vi "log analysis_gps.vi"() -> ()   [LabVIEW 2018] (continued)
10.7036,22.3000,-0.1718,0.2091,0.0001,-1.383604006,1.084294313,122.725543764,0.4496,0.3001,0.5813,0.1247,0.1017,0.0764,0.1414,0.1471,4.9509,0f000001,0*50e8e3f0\n\t", "DUALANTENNAHEADINGA,USB3,0,49.0,FINESTEERING,2107,282338.100,02000000,d426,15824;SOL_COMPUTED,L1_FLOAT,-1.000000000,82.313255310,23.154996872,0.0,360.000000000,180.000000000,\"631T\",16,5,5,3,04,00,20,01*91a11998\n\t", "DUALANTENNAHEADINGA,USB3,0,50.5,FINESTEERING,2107,282339.100,02008000,d426,15824;INSUFFICIENT_OBS,NONE,0.000000000,0.000000000,0.000000000,0.0,0.000000000,0.000000000,\"\",0,0,0,0,00,00,00,00*9d87d1bd\n\t", "INSPVAXA,USB3,0,52.0,FINESTEERING,2107,282339.650,02008000,471d,15824;INS_ALIGNMENT_COMPLETE,INS_RTKFIXED,37.37060410309,126.72431070985,10.7187,22.3000,-0.1560,0.2044,-0.0028,-0.834208822,1.087221031,121.798208463,0.4988,0.3371,0.6091,0.1298,0.1043,0.0790,0.1415,0.1476,4.9532,0f000001,0*1343af04\n\t", "DUALANTENNAHEADINGA,USB3,0,50.5,FINESTEERING,2107,282340.100,02008000,d426,15824;INSUFFICIENT_OBS,NONE,0.000000000,0.000000000,0.000000000,0.0,0.000000000,0.000000000,\"\",0,0,0,0,00,00,00,00*7b9cfbae\n\t", "DUALANTENNAHEADINGA,USB3,0,50.5,FINESTEERING,2107,282340.600,02008000,d426,15824;INSUFFICIENT_OBS,NONE,0.000000000,0.000000000,0.000000000,0.0,0.000000000,0.000000000,\"\",0,0,0,0,00,00,00,00*d2d79b9f\n\t", "DUALANTENNAHEADINGA,USB3,0,50.5,FINESTEERING,2107,282341.100,02008000,d426,15824;SOL_COMPUTED,NARROW_FLOAT,-1.000000000,114.279808044,-67.503875732,0.0,360.000000000,180.000000000,\"631T\",19,7,7,5,04,00,20,03*2721f886\n\t", "INSPVAXA,USB3,0,51.0,FINESTEERING,2107,282341.650,02008000,471d,15824;INS_ALIGNMENT_COMPLETE,INS_RTKFIXED,37.37060132873,126.72431550625,10.7234,22.3000,-0.1474,0.2047,-0.0035,-0.652632688,1.321187419,121.044830235,0.4988,0.3371,0.6091,0.1298,0.1043,0.0790,0.1415,0.1476,4.9532,0f000001,0*64211db3\n\t", "DUALANTENNAHEADINGA,USB3,0,51.0,FINESTEERING,2107,282342.100,02008000,d426,15824;INSUFFICIENT_OBS,NONE,0.000000000,0.000000000,0.000000000,0.0,0.000000000,0.000000000,\"\",0,0,0,0,00,00,00,00*1fd29d28\n\t", "DUALANTENNAHEADINGA,USB3,0,53.0,FINESTEERING,2107,282342.600,02008000,d426,15824;INSUFFICIENT_OBS,NONE,0.000000000,0.000000000,0.000000000,0.0,0.000000000,0.000000000,\"\",0,0,0,0,00,00,00,00*2c3b97de\n\t", "INSPVAXA,USB3,0,54.0,FINESTEERING,2107,282344.150,02000000,471d,15824;INS_ALIGNMENT_COMPLETE,INS_RTKFIXED,37.37059762700,126.72432213612,10.7457,22.3000,-0.1412,0.2163,0.0072,-0.887257962,1.775723186,120.744197339,0.5693,0.3802,0.6775,0.1345,0.1064,0.0820,0.1423,0.1482,4.9577,0f000001,0*eda97082\n\t", "INSPVAXA,USB3,0,54.0,FINESTEERING,2107,282344.650,02000000,471d,15824;INS_ALIGNMENT_COMPLETE,INS_RTKFIXED,37.37059696338,126.72432331213,10.7485,22.3000,-0.1428,0.2163,0.0073,-0.851471886,1.782877792,120.701591584,0.5693,0.3802,0.6775,0.1345,0.1064,0.0820,0.1423,0.1482,4.9577,0f000001,0*59042419\n\t", "INSPVAXA,USB3,0,55.5,FINESTEERING,2107,282345.150,02000000,471d,15824;INS_ALIGNMENT_COMPLETE,INS_RTKFIXED,37.37059621025,126.72432460307,10.7527,22.3000,-0.1388,0.2123,-0.0024,-0.823739386,1.527099287,120.736340769,0.5930,0.3895,0.7245,0.1352,0.1094,0.0826,0.1432,0.1486,4.9599,0f000001,0*b8434a6e\n\t", "DUALANTENNAHEADINGA,USB3,0,55.5,FINESTEERING,2107,282345.600,02000000,d426,15824;SOL_COMPUTED,L1_FLOAT,-1.000000000,162.531326294,-26.929321289,0.0,360.000000000,180.000000000,\"631T\",14,5,5,5,04,00,20,03*11a6b9e7\n\t", "INSPVAXA,USB3,0,51.0,FINESTEERING,2107,282346.650,02000000,471d,15824;INS_ALIGNMENT_COMPLETE,INS_RTKFIXED,37.37059354728,126.72432896514,10.7808,22.3000,-0.1593,0.2217,0.0028,-1.002740448,1.844752135,120.714031734,0.5188,0.3373,0.6687,0.1274,0.1044,0.0789,0.1425,0.1477,4.9597,0f000001,0*e05fc804\n\t", "INSPVAXA,USB3,0,53.5,FINESTEERING,2107,282347.150,02000000,471d,15824;INS_ALIGNMENT_COMPLETE,INS_RTKFIXED,37.37059272987,126.72433032061,10.7898,22.3000,-0.1653,0.2242,0.0071,-0.929787730,1.969126330,120.702008757,0.4813,0.3140,0.6303,0.1252,0.1036,0.0771,0.1422,0.1473,4.9596,0f000001,0*9ccf88c1\n\t", "INSPVAXA,USB3,0,53.5,FINESTEERING,2107,282347.650,02000000,471d,15824;INS_ALIGNMENT_COMPLETE,INS_RTKFIXED,37.37059194697,126.72433163028,10.7970,22.3000,-0.1569,0.2242,0.0124,-0.943778320,2.029286352,120.707003262,0.4813,0.3140,0.6303,0.1252,0.1036,0.0771,0.1422,0.1473,4.9596,0f000001,0*cfe1604c\n\t", "INSPVAXA,USB3,0,51.5,FINESTEERING,2107,282348.650,02000000,471d,15824;INS_ALIGNMENT_COMPLETE,INS_RTKFIXED,37.37059036777,126.72433430477,10.8134,22.3000,-0.1636,0.2313,0.0075,-1.033266783,1.805769894,120.739350596,0.4628,0.3038,0.6031,0.1249,0.1034,0.0763,0.1419,0.1472,4.9599,0f000001,0*467420a2\n\t", "INSPVAXA,USB3,0,51.5,FINESTEERING,2107,282349.650,02000000,471d,15824;INS_ALIGNMENT_COMPLETE,INS_RTKFIXED,37.37058879299,126.72433694056,10.8279,22.3000,-0.1661,0.2333,0.0109,-1.186914388,1.463198419,120.784374977,0.4532,0.2999,0.5832,0.1247,0.1026,0.0761,0.1414,0.1469,4.9608,0f000001,0*9616f401\n\t", "INSPVAXA,USB3,0,52.5,FINESTEERING,2107,282350.150,02000000,471d,15824;INS_ALIGNMENT_COMPLETE,INS_RTKFIXED,37.37058797901,126.72433827202,10.8352,22.3000,-0.1763,0.2301,0.0086,-1.055570073,1.334834507,120.760295852,0.4480,0.2986,0.5686,0.1241,0.1011,0.0762,0.1408,0.1465,4.9619,0f000001,0*f726bccb\n\t", "INSPVAXA,USB3,0,52.5,FINESTEERING,2107,282350.650,02000000,471d,15824;INS_ALIGNMENT_COMPLETE,INS_RTKFIXED,37.37058716740,126.72433957539,10.8417,22.3000,-0.1740,0.2264,0.0121,-0.872298800,1.208067122,120.805643727,0.4480,0.2986,0.5686,0.1241,0.1011,0.0762,0.1408,0.1465,4.9619,0f000001,0*1bc0a6ef\n\t", "INSPVAXA,USB3,0,53.5,FINESTEERING,2107,282351.150,02000000,471d,15824;INS_ALIGNMENT_COMPLETE,INS_RTKFIXED,37.37058636021,126.72434089175,10.8474,22.3000,-0.1737,0.2293,0.0134,-0.911883774,0.960654196,120.863326137,0.4480,0.2986,0.5686,0.1241,0.1011,0.0762,0.1408,0.1465,4.9619,0f000001,0*f3ef71b8\n\t", "INSPVAXA,USB3,0,53.5,FINESTEERING,2107,282351.650,02000000,471d,15824;INS_ALIGNMENT_COMPLETE,INS_RTKFIXED,37.37058558937,126.72434215471,10.8538,22.3000,-0.1759,0.2200,0.0154,-0.934777564,1.004148344,120.872982319,0.4480,0.2986,0.5686,0.1241,0.1011,0.0762,0.1408,0.1465,4.9619,0f000001,0*31170c67\n\t", "INSPVAXA,USB3,0,53.0,FINESTEERING,2107,282352.150,02000000,471d,15824;INS_ALIGNMENT_COMPLETE,INS_RTKFIXED,37.37058479579,126.72434342427,10.8616,22.3000,-0.1887,0.2204,0.0143,-0.790488347,0.999839674,120.821997376,0.4480,0.2986,0.5686,0.1241,0.1011,0.0762,0.1408,0.1465,4.9619,0f000001,0*9c9f2292\n\t", "INSPVAXA,USB3,0,53.0,FINESTEERING,2107,282352.650,02000000,471d,15824;INS_ALIGNMENT_COMPLETE,INS_RTKFIXED,37.37058401212,126.72434466825,10.8699,22.3000,-0.1898,0.2115,0.0109,-0.691065939,1.126816556,120.801550290,0.4480,0.2986,0.5686,0.1241,0.1011,0.0762,0.1408,0.1465,4.9619,0f000001,0*dfeeaeca\n\t", "INSPVAXA,USB3,0,54.5,FINESTEERING,2107,282353.150,02000000,471d,15824;INS_ALIGNMENT_COMPLETE,INS_RTKFIXED,37.37058321062,126.72434596398,10.8773,22.3000,-0.1742,0.2198,0.0094,-0.675574846,1.167497971,120.763135201,0.5451,0.3682,0.6457,0.1338,0.1065,0.0809,0.1421,0.1478,4.9659,0f000001,0*3ed9f220\n\t", "INSPVAXA,USB3,0,54.5,FINESTEERING,2107,282353.650,02000000,471d,15824;INS_ALIGNMENT_COMPLETE,INS_RTKFIXED,37.37058240140,126.72434728277,10.8821,22.3000,-0.1762,0.2174,0.0139,-0.658240149,1.464684464,120.605097651,0.5451,0.3682,0.6457,0.1338,0.1065,0.0809,0.1421,0.1478,4.9659,0f000001,0*55075841\n\t", "INSPVAXA,USB3,0,46.0,FINESTEERING,2107,282354.150,02000000,471d,15824;INS_ALIGNMENT_COMPLETE,INS_RTKFIXED,37.37058158517,126.72434860573,10.8883,22.3000,-0.1761,0.2236,0.0096,-0.460607316,1.517794635,120.410253165,0.4992,0.3307,0.6168,0.1257,0.0997,0.0788,0.1413,0.1466,4.9674,0f000001,0*75609bcc\n\t", "INSPVAXA,USB3,0,46.0,FINESTEERING,2107,282354.650,02000000,471d,15824;INS_ALIGNMENT_COMPLETE,INS_RTKFIXED,37.37058081600,126.72434991701,10.8934,22.3000,-0.1786,0.2176,0.0091,-0.549619810,1.573012469,120.242291746,0.4992,0.3307,0.6168,0.1257,0.0997,0.0788,0.1413,0.1466,4.9674,0f000001,0*21503aba\n\t", "INSPVAXA,USB3,0,52.5,FINESTEERING,2107,282355.150,02000000,471d,15824;INS_ALIGNMENT_COMPLETE,INS_RTKFIXED,37.37058003617,126.72435122954,10.8990,22.3000,-0.1704,0.2109,0.0104,-0.583465901,1.528119993,119.981024145,0.4739,0.3119,0.5957,0.1220,0.0977,0.0777,0.1410,0.1462,4.9689,0f000001,0*126057fe\n\t", "INSPVAXA,USB3,0,52.5,FINESTEERING,2107,282355.650,02000000,471d,15824;INS_ALIGNMENT_COMPLETE,INS_RTKFIXED,37.37057924767,126.72435254533,10.9045,22.3000,-0.1778,0.2238,0.0059,-0.556149260,1.423178014,119.692620317,0.4739,0.3119,0.5957,0.1220,0.0977,0.0777,0.1410,0.1462,4.9689,0f000001,0*50fd9e16\n\t", "INSPVAXA,USB3,0,50.5,FINESTEERING,2107,282356.150,02000000,471d,15824;INS_ALIGNMENT_COMPLETE,INS_RTKFIXED,37.37057847739,126.72435384843,10.9119,22.3000,-0.1686,0.2211,0.0250,-0.610838091,1.352028935,119.375016734,0.4594,0.3023,0.5798,0.1203,0.0972,0.0771,0.1409,0.1459,4.9699,0f000001,0*f72577eb\n\t", "INSPVAXA,USB3,0,50.5,FINESTEERING,2107,282356.650,02000000,471d,15824;INS_ALIGNMENT_COMPLETE,INS_RTKFIXED,37.37057772160,126.72435517265,10.9178,22.3000,-0.1723,0.2271,0.0230,-0.636591933,1.172282791,119.120900603,0.4594,0.3023,0.5798,0.1203,0.0972,0.0771,0.1409,0.1459,4.9699,0f000001,0*423d8117\n\t", "INSPVAXA,USB3,0,52.0,FINESTEERING,2107,282357.150,02000000,471d,15824;INS_ALIGNMENT_COMPLETE,INS_RTKFIXED,37.37057699183,126.72435647012,10.9247,22.3000,-0.1655,0.2123,0.0266,-0.635674987,1.199232102,118.840756157,0.4503,0.2976,0.5676,0.1194,0.0970,0.0768,0.1408,0.1458,4.9705,0f000001,0*6596f8d2\n\t", "INSPVAXA,USB3,0,52.0,FINESTEERING,2107,282357.650,02000000,471d,15824;INS_ALIGNMENT_COMPLETE,INS_RTKFIXED,37.37057627543,126.72435778684,10.9314,22.3000,-0.1654,0.2174,0.0126,-0.648643975,1.318562977,118.602215065,0.4503,0.2976,0.5676,0.1194,0.0970,0.0768,0.1408,0.1458,4.9705,0f000001,0*56e0c8f4\n\t", "INSPVAXA,USB3,0,49.0,FINESTEERING,2107,282358.150,02000000,471d,15824;INS_ALIGNMENT_COMPLETE,INS_RTKFIXED,37.37057556621,126.72435909816,10.9380,22.3000,-0.1614,0.2140,0.0160,-0.816236405,1.456902249,118.427735128,0.4453,0.2956,0.5586,0.1188,0.0967,0.0767,0.1406,0.1456,4.9710,0f000001,0*b637b657\n\t", "INSPVAXA,USB3,0,49.0,FINESTEERING,2107,282358.650,02000000,471d,15824;INS_ALIGNMENT_COMPLETE,INS_RTKFIXED,37.37057483953,126.72436042274,10.9431,22.3000,-0.1620,0.2072,0.0216,-0.840006247,1.481756490,118.251827857,0.4453,0.2956,0.5586,0.1188,0.0967,0.0767,0.1406,0.1456,4.9710,0f000001,0*14500fa5\n\t", "INSPVAXA,USB3,0,50.0,FINESTEERING,2107,282359.150,02000000,471d,15824;INS_ALIGNMENT_COMPLETE,INS_RTKFIXED,37.37057411290,126.72436171376,10.9480,22.3000,-0.1710,0.2086,0.0288,-0.732849795,1.756620997,118.132387326,0.4424,0.2949,0.5520,0.1182,0.0959,0.0768,0.1404,0.1455,4.9710,0f000001,0*33ffa9dc\n\t", "INSPVAXA,USB3,0,50.0,FINESTEERING,2107,282359.650,02000000,471d,15824;INS_ALIGNMENT_COMPLETE,INS_RTKFIXED,37.37057338322,126.72436305467,10.9529,22.3000,-0.1728,0.2229,0.0180,-0.801068797,1.536454287,118.115818478,0.4424,0.2949,0.5520,0.1182,0.0959,0.0768,0.1404,0.1455,4.9710,0f000001,0*c3454afa\n\t", "INSPVAXA,USB3,0,48.5,FINESTEERING,2107,282360.150,02000000,471d,15824;INS_ALIGNMENT_COMPLETE,INS_RTKFIXED,37.37057265059,126.72436438219,10.9582,22.3000,-0.1754,0.2257,0.0186,-0.842848206,1.417409471,118.070069819,0.4412,0.2945,0.5472,0.1174,0.0950,0.0769,0.1402,0.1453,4.9710,0f000001,0*6a16ee00\n\t", "INSPVAXA,USB3,0,48.5,FINESTEERING,2107,282360.650,02000000,471d,15824;INS_ALIGNMENT_COMPLETE,INS_RTKFIXED,37.37057191747,126.72436570845,10.9626,22.3000,-0.1784,0.2288,0.0199,-0.831650114,1.387719615,118.066694933,0.4412,0.2945,0.5472,0.1174,0.0950,0.0769,0.1402,0.1453,4.9710,0f000001,0*684747fc\n\t", "INSPVAXA,USB3,0,48.0,FINESTEERING,2107,282361.650,02000000,471d,15824;INS_ALIGNMENT_COMPLETE,INS_RTKFIXED,37.37057042530,126.72436839921,10.9712,22.3000,-0.1758,0.2244,0.0130,-0.782174586,1.064389692,118.205019127,0.4403,0.2942,0.5440,0.1166,0.0940,0.0770,0.1401,0.1452,4.9712,0f000001,0*a289776d\n\t", "INSPVAXA,USB3,0,52.0,FINESTEERING,2107,282362.150,02000000,471d,15824;INS_ALIGNMENT_COMPLETE,INS_RTKFIXED,37.37056968661,126.72436971158,10.9754,22.3000,-0.1789,0.2227,0.0149,-0.712007512,1.145542222,118.217293959,0.4394,0.2937,0.5418,0.1158,0.0932,0.0771,0.1400,0.1450,4.9721,0f000001,0*3affd318\n\t", "INSPVAXA,USB3,0,52.0,FINESTEERING,2107,282362.650,02000000,471d,15824;INS_ALIGNMENT_COMPLETE,INS_RTKFIXED,37.37056893906,126.72437106065,10.9790,22.3000,-0.1744,0.2169,0.0071,-0.647011256,1.079419362,118.301292650,0.4394,0.2937,0.5418,0.1158,0.0932,0.0771,0.1400,0.1450,4.9721,0f000001,0*1e26d504\n\t", "INSPVAXA,USB3,0,52.5,FINESTEERING,2107,282363.150,02000000,471d,15824;INS_ALIGNMENT_COMPLETE,INS_RTKFIXED,37.37056818219,126.72437236922,10.9848,22.3000,-0.1880,0.2251,0.0164,-0.692024407,1.031121061,118.296623598,0.4394,0.2937,0.5418,0.1158,0.0932,0.0771,0.1400,0.1450,4.9721,0f000001,0*fbc0c197\n\t", "INSPVAXA,USB3,0,52.5,FINESTEERING,2107,282363.650,02000000,471d,15824;INS_ALIGNMENT_COMPLETE,INS_RTKFIXED,37.37056736764,126.72437362581,10.9943,22.3000,-0.1838,0.2175,0.0187,-0.622586307,1.194821727,118.320117324,0.4394,0.2937,0.5418,0.1158,0.0932,0.0771,0.1400,0.1450,4.9721,0f000001,0*9ae06ad3\n\t", "INSPVAXA,USB3,0,46.5,FINESTEERING,2107,282364.150,02000000,471d,15824;INS_ALIGNMENT_COMPLETE,INS_RTKFIXED,37.37056657190,126.72437491440,11.0023,22.3000,-0.1853,0.2142,0.0193,-0.566287022,1.525613258,118.367713694,0.4907,0.3307,0.5859,0.1218,0.0978,0.0797,0.1410,0.1460,4.9751,0f000001,0*d0324f7d\n\t", "INSPVAXA,USB3,0,46.5,FINESTEERING,2107,282364.650,02000000,471d,15824;INS_ALIGNMENT_COMPLETE,INS_RTKFIXED,37.37056585214,126.72437630982,11.0047,22.3000,-0.1882,0.2248,0.0125,-0.569851294,1.528591804,118.479722218,0.4907,0.3307,0.5859,0.1218,0.0978,0.0797,0.1410,0.1460,4.9751,0f000001,0*9a426144\n\t", "INSPVAXA,USB3,0,48.5,FINESTEERING,2107,282365.650,02000000,471d,15824;INS_ALIGNMENT_COMPLETE,INS_RTKFIXED,37.37056440793,126.72437904086,11.0071,22.3000,-0.1949,0.2319,0.0130,-0.541846536,1.457071221,118.616213426,0.4699,0.3127,0.5753,0.1175,0.0943,0.0785,0.1406,0.1454,4.9762,0f000001,0*40288813\n\t", "INSPVAXA,USB3,0,51.0,FINESTEERING,2107,282366.650,02000000,471d,15824;INS_ALIGNMENT_COMPLETE,INS_RTKFIXED,37.37056291329,126.72438179261,11.0096,22.3000,-0.1917,0.2323,0.0080,-0.472728145,0.808367431,118.811459279,0.4569,0.3025,0.5669,0.1155,0.0932,0.0778,0.1406,0.1452,4.9769,0f000001,0*4a7ebce1\n\t", "INSPVAXA,USB3,0,52.5,FINESTEERING,2107,282367.150,02000000,471d,15824;INS_ALIGNMENT_COMPLETE,INS_RTKFIXED,37.37056215950,126.72438315251,11.0104,22.3000,-0.1905,0.2375,-0.0008,-0.383174802,0.623906770,118.905218595,0.4483,0.2967,0.5601,0.1147,0.0932,0.0773,0.1406,0.1452,4.9782,0f000001,0*ea495475\n\t", "INSPVAXA,USB3,0,52.5,FINESTEERING,2107,282367.650,02000000,471d,15824;INS_ALIGNMENT_COMPLETE,INS_RTKFIXED,37.37056140665,126.72438451966,11.0108,22.3000,-0.1856,0.2294,0.0072,-0.390392792,0.506918836,119.017967456,0.4483,0.2967,0.5601,0.1147,0.0932,0.0773,0.1406,0.1452,4.9782,0f000001,0*a0cb1e22\n\t", "INSPVAXA,USB3,0,51.0,FINESTEERING,2107,282368.150,02000000,471d,15824;INS_ALIGNMENT_COMPLETE,INS_RTKFIXED,37.37056062590,126.72438588956,11.0109,22.3000,-0.1908,0.2384,0.0056,-0.245023334,0.482634279,119.176381690,0.4426,0.2937,0.5546,0.1146,0.0935,0.0770,0.1406,0.1452,4.9797,0f000001,0*61c8f471\n\t", "INSPVAXA,USB3,0,49.0,FINESTEERING,2107,282370.150,02000000,471d,15824;INS_ALIGNMENT_COMPLETE,INS_RTKFIXED,37.37055758372,126.72439118773,11.0127,22.3000,-0.1993,0.2333,0.0205,-0.126523860,1.017645385,119.745065881,0.4369,0.2920,0.5469,0.1146,0.0935,0.0767,0.1404,0.1452,4.9818,0f000001,0*3c99dcc1\n\t", "INSPVAXA,USB3,0,49.0,FINESTEERING,2107,282370.650,02000000,471d,15824;INS_ALIGNMENT_COMPLETE,INS_RTKFIXED,37.37055683678,126.72439251585,11.0116,22.3000,-0.1882,0.2280,0.0157,-0.028794832,1.243937117,119.855600640,0.4369,0.2920,0.5469,0.1146,0.0935,0.0767,0.1404,0.1452,4.9818,0f000001,0*7496fdf6\n\t", "INSPVAXA,USB3,0,50.0,FINESTEERING,2107,282371.150,02000000,471d,15824;INS_ALIGNMENT_COMPLETE,INS_RTKFIXED,37.37055608815,126.72439385420,11.0119,22.3000,-0.1947,0.2327,0.0119,-0.172585460,1.434683423,119.971021632,0.4362,0.2920,0.5445,0.1145,0.0933,0.0767,0.1403,0.1451,4.9828,0f000001,0*21210484\n\t", "INSPVAXA,USB3,0,51.5,FINESTEERING,2107,282372.150,02000000,471d,15824;INS_ALIGNMENT_COMPLETE,INS_RTKFIXED,37.37055456936,126.72439651011,11.0164,22.3000,-0.1955,0.2409,0.0111,-0.219662540,1.523066088,120.209141844,0.4362,0.2922,0.5426,0.1144,0.0930,0.0767,0.1402,0.1451,4.9843,0f000001,0*f3fda870\n\t", "INSPVAXA,USB3,0,51.5,FINESTEERING,2107,282372.650,02000000,471d,15824;INS_ALIGNMENT_COMPLETE,INS_RTKFIXED,37.37055382453,126.72439783430,11.0178,22.3000,-0.1964,0.2384,0.0010,-0.282113578,1.525554977,120.284642738,0.4362,0.2922,0.5426,0.1144,0.0930,0.0767,0.1402,0.1451,4.9843,0f000001,0*1248182f\n\t", "INSPVAXA,USB3,0,48.5,FINESTEERING,2107,282374.150,02000000,471d,15824;INS_ALIGNMENT_COMPLETE,INS_RTKFIXED,37.37055158865,126.72440177016,11.0240,22.3000,-0.1992,0.2398,-0.0010,-0.425522010,1.592578563,120.559312340,0.4364,0.2923,0.5406,0.1141,0.0924,0.0768,0.1401,0.1450,4.9874,0f000001,0*101c3bdb\n\t", "INSPVAXA,USB3,0,51.0,FINESTEERING,2107,282375.150,02000000,471d,15824;INS_ALIGNMENT_COMPLETE,INS_RTKFIXED,37.37055007830,126.72440434973,11.0274,22.3000,-0.1945,0.2378,0.0125,-0.376290277,1.647280363,120.637326967,0.4364,0.2922,0.5400,0.1139,0.0922,0.0768,0.1401,0.1450,4.9889,0f000001,0*67dcfdd6\n\t", "INSPVAXA,USB3,0,50.5,FINESTEERING,2107,282376.150,02000000,471d,15824;INS_ALIGNMENT_COMPLETE,INS_RTKFIXED,37.37054852803,126.72440700509,11.0323,22.3000,-0.1988,0.2410,0.0047,-0.545420611,1.322594282,120.751487308,0.4364,0.2922,0.5400,0.1139,0.0922,0.0768,0.1401,0.1450,4.9889,0f000001,0*a32cf91e\n\t", "INSPVAXA,USB3,0,56.0,FINESTEERING,2107,282377.150,02000000,471d,15824;INS_ALIGNMENT_COMPLETE,INS_RTKFIXED,37.37054676587,126.72440967582,11.0390,22.3000,-0.1999,0.2394,0.0134,-0.643659159,1.057296684,120.890681987,0.4364,0.2922,0.5400,0.1139,0.0922,0.0768,0.1401,0.1450,4.9889,0f000001,0*19d68dee\n\t", "INSPVAXA,USB3,0,51.5,FINESTEERING,2107,282380.150,02000000,471d,15824;INS_ALIGNMENT_COMPLETE,INS_RTKFIXED,37.37054231634,126.72441746453,11.0545,22.3000,-0.1950,0.2290,0.0101,-0.779433924,1.099591646,120.976695611,0.4675,0.3093,0.5930,0.1184,0.0970,0.0772,0.1414,0.1460,4.9947,0f000001,0*af9d06d5\n\t", "INSPVAXA,USB3,0,53.0,FINESTEERING,2107,282396.200,02000000,471d,15824;INS_ALIGNMENT_COMPLETE,INS_RTKFIXED,37.37051727534,126.72445893614,11.2346,22.3000,-0.2149,0.2448,0.0105,-0.230381953,1.670919034,121.706042723,0.4454,0.2945,0.5444,0.1167,0.0933,0.0771,0.1396,0.1448,5.0169,0f000001,0*e3a105a8\n\t", "INSPVAXA,USB3,0,52.5,FINESTEERING,2107,282399.700,02000000,471d,15824;INS_ALIGNMENT_COMPLETE,INS_RTKFIXED,37.37051173912,126.72446803450,11.2629,22.3000,-0.2157,0.2432,0.0104,-0.126649868,1.183808073,120.810959551,0.4494,0.2941,0.5444,0.1155,0.0921,0.0775,0.1396,0.1447,5.0208,0f000001,0*57a15611\n\t", "INSPVAXA,USB3,0,51.5,FINESTEERING,2107,282400.200,02000000,471d,15824;INS_ALIGNMENT_COMPLETE,INS_RTKFIXED,37.37051098079,126.72446931042,11.2663,22.3000,-0.2068,0.2423,0.0047,-0.194058602,1.122857123,120.589823258,0.4487,0.2937,0.5447,0.1150,0.0920,0.0775,0.1397,0.1447,5.0216,0f000001,0*c9fba93a\n\t", "INSPVAXA,USB3,0,51.5,FINESTEERING,2107,282400.700,02000000,471d,15824;INS_ALIGNMENT_COMPLETE,INS_RTKFIXED,37.37051023771,126.72447057615,11.2691,22.3000,-0.2018,0.2421,0.0003,-0.178083607,1.252069735,120.254195677,0.4487,0.2937,0.5447,0.1150,0.0920,0.0775,0.1397,0.1447,5.0216,0f000001,0*c019cdcb\n\t", "INSPVAXA,USB3,0,52.0,FINESTEERING,2107,282402.700,02000000,471d,15824;INS_ALIGNMENT_COMPLETE,INS_RTKFIXED,37.37050732665,126.72447567900,11.2840,22.3000,-0.1846,0.2304,0.0147,-0.197464539,1.720744587,119.244672502,0.4474,0.2933,0.5456,0.1143,0.0919,0.0775,0.1398,0.1447,5.0227,0f000001,0*ef6b078e\n\t", "INSPVAXA,USB3,0,51.0,FINESTEERING,2107,282403.700,02000000,471d,15824;INS_ALIGNMENT_COMPLETE,INS_RTKFIXED,37.37050587454,126.72447826035,11.2883,22.3000,-0.1895,0.2228,0.0117,-0.041463128,1.413686081,119.013719695,0.4466,0.2931,0.5458,0.1142,0.0920,0.0774,0.1398,0.1448,5.0238,0f000001,0*aa5be0c8\n\t", "INSPVAXA,USB3,0,53.0,FINESTEERING,2107,282405.200,02000000,471d,15824;INS_ALIGNMENT_COMPLETE,INS_RTKFIXED,37.37050369833,126.72448216938,11.2960,22.3000,-0.1948,0.2280,0.0025,-0.062260759,1.020577864,118.930310663,0.4445,0.2927,0.5458,0.1142,0.0920,0.0773,0.1398,0.1448,5.0258,0f000001,0*8918fe41\n\t", "INSPVAXA,USB3,0,49.0,FINESTEERING,2107,282406.200,02000000,471d,15824;INS_ALIGNMENT_COMPLETE,INS_RTKFIXED,37.37050223457,126.72448478438,11.2989,22.3000,-0.1940,0.2271,0.0004,0.403911528,1.100287176,119.003406163,0.4431,0.2925,0.5454,0.1141,0.0922,0.0772,0.1398,0.1448,5.0266,0f000001,0*9acaefa2\n\t", "INSPVAXA,USB3,0,49.0,FINESTEERING,2107,282406.700,02000000,471d,15824;INS_ALIGNMENT_COMPLETE,INS_RTKFIXED,37.37050154645,126.72448605087,11.3007,22.3000,-0.1906,0.2211,-0.0024,0.198399759,1.155504209,119.019429949,0.4431,0.2925,0.5454,0.1141,0.0922,0.0772,0.1398,0.1448,5.0266,0f000001,0*2b05d55f\n\t", "INSPVAXA,USB3,0,49.5,FINESTEERING,2107,282407.200,02000000,471d,15824;INS_ALIGNMENT_COMPLETE,INS_RTKFIXED,37.37050082511,126.72448737364,11.3024,22.3000,-0.1843,0.2252,0.0031,0.001432132,1.154226626,118.999213590,0.4420,0.2924,0.5450,0.1140,0.0921,0.0771,0.1398,0.1448,5.0273,0f000001,0*acf3bb7b\n\t", "INSPVAXA,USB3,0,49.5,FINESTEERING,2107,282407.700,02000000,471d,15824;INS_ALIGNMENT_COMPLETE,INS_RTKFIXED,37.37050009749,126.72448866196,11.3047,22.3000,-0.1922,0.2264,0.0013,0.031954534,1.373571777,119.029897417,0.4420,0.2924,0.5450,0.1140,0.0921,0.0771,0.1398,0.1448,5.0273,0f000001,0*4feaee25\n\t", "INSPVAXA,USB3,0,49.5,FINESTEERING,2107,282408.700,02000000,471d,15824;INS_ALIGNMENT_COMPLETE,INS_RTKFIXED,37.37049862952,126.72449128459,11.3098,22.3000,-0.1866,0.2253,0.0102,0.047127376,1.614716400,119.167288999,0.4410,0.2922,0.5445,0.1140,0.0921,0.0770,0.1398,0.1448,5.0281,0f000001,0*196c2f22\n\t", "INSPVAXA,USB3,0,47.5,FINESTEERING,2107,282409.200,02000000,471d,15824;INS_ALIGNMENT_COMPLETE,INS_RTKFIXED,37.37049789341,126.72449262767,11.3125,22.3000,-0.1999,0.2359,0.0079,-0.178457330,1.548416838,119.244672995,0.4408,0.2923,0.5442,0.1140,0.0922,0.0770,0.1398,0.1448,5.0295,0f000001,0*fefe7bbe\n\t", "INSPVAXA,USB3,0,49.0,FINESTEERING,2107,282410.700,02000000,471d,15824;INS_ALIGNMENT_COMPLETE,INS_RTKFIXED,37.37049566854,126.72449665280,11.3239,22.3000,-0.1868,0.2363,0.0016,-0.505574846,1.345277164,119.533703259,0.4402,0.2922,0.5436,0.1139,0.0922,0.0769,0.1398,0.1447,5.0311,0f000001,0*6012c6b0\n\t", "INSPVAXA,USB3,0,50.0,FINESTEERING,2107,282411.200,02000000,471d,15824;INS_ALIGNMENT_COMPLETE,INS_RTKFIXED,37.37049487353,126.72449799751,11.3279,22.3000,-0.1792,0.2394,0.0156,-0.401695145,1.333527826,119.633898753,0.4402,0.2922,0.5436,0.1139,0.0922,0.0769,0.1398,0.1447,5.0311,0f000001,0*2fc42002\n\t", "INSPVAXA,USB3,0,50.0,FINESTEERING,2107,282411.700,02000000,471d,15824;INS_ALIGNMENT_COMPLETE,INS_RTKFIXED,37.37049401462,126.72449935015,11.3332,22.3000,-0.1865,0.2337,0.0135,-0.484899234,1.283665048,119.740703059,0.4402,0.2922,0.5436,0.1139,0.0922,0.0769,0.1398,0.1447,5.0311,0f000001,0*1d33eb73\n\t", "INSPVAXA,USB3,0,45.5,FINESTEERING,2107,282412.200,02000000,471d,15824;INS_ALIGNMENT_COMPLETE,INS_RTKFIXED,37.37049319930,126.72450071545,11.3390,22.3000,-0.1883,0.2399,0.0132,-0.511269715,1.109019547,119.856142336,0.4907,0.3298,0.5890,0.1210,0.0979,0.0793,0.1408,0.1457,5.0340,0f000001,0*b0282710\n\t", "INSPVAXA,USB3,0,45.5,FINESTEERING,2107,282412.700,02000000,471d,15824;INS_ALIGNMENT_COMPLETE,INS_RTKFIXED,37.37049251112,126.72450203682,11.3445,22.3000,-0.1885,0.2438,0.0204,-0.533735812,1.097181007,119.915108239,0.4907,0.3298,0.5890,0.1210,0.0979,0.0793,0.1408,0.1457,5.0340,0f000001,0*9a141504\n\t", "INSPVAXA,USB3,0,46.5,FINESTEERING,2107,282413.200,02000000,471d,15824;INS_ALIGNMENT_COMPLETE,INS_RTKFIXED,37.37049180169,126.72450336418,11.3490,22.3000,-0.1814,0.2477,0.0198,-0.567250496,1.161668497,119.990441604,0.4687,0.3125,0.5782,0.1173,0.0947,0.0780,0.1403,0.1452,5.0347,0f000001,0*907c6878\n\t", "INSPVAXA,USB3,0,46.5,FINESTEERING,2107,282413.700,02000000,471d,15824;INS_ALIGNMENT_COMPLETE,INS_RTKFIXED,37.37049106798,126.72450467966,11.3532,22.3000,-0.1907,0.2386,0.0196,-0.535844359,1.216959402,120.030591907,0.4687,0.3125,0.5782,0.1173,0.0947,0.0780,0.1403,0.1452,5.0347,0f000001,0*639bb67e\n\t", "INSPVAXA,USB3,0,51.5,FINESTEERING,2107,282414.200,02000000,471d,15824;INS_ALIGNMENT_COMPLETE,INS_RTKFIXED,37.37049032617,126.72450602273,11.3581,22.3000,-0.1924,0.2499,0.0107,-0.616512696,1.220090147,120.041431319,0.4551,0.3027,0.5696,0.1158,0.0939,0.0773,0.1402,0.1450,5.0349,0f000001,0*41bc56e6\n\t", "INSPVAXA,USB3,0,51.5,FINESTEERING,2107,282414.700,02000000,471d,15824;INS_ALIGNMENT_COMPLETE,INS_RTKFIXED,37.37048957210,126.72450735141,11.3626,22.3000,-0.1833,0.2491,0.0031,-0.413726161,1.254488863,120.030297293,0.4551,0.3027,0.5696,0.1158,0.0939,0.0773,0.1402,0.1450,5.0349,0f000001,0*52de2f77\n\t", "INSPVAXA,USB3,0,53.0,FINESTEERING,2107,282415.200,02000000,471d,15824;INS_ALIGNMENT_COMPLETE,INS_RTKFIXED,37.37048882282,126.72450867783,11.3669,22.3000,-0.1974,0.2488,-0.0050,-0.369163180,1.275233001,120.010997524,0.4468,0.2975,0.5625,0.1152,0.0938,0.0768,0.1401,0.1449,5.0346,0f000001,0*63e54e05\n\t", "INSPVAXA,USB3,0,53.0,FINESTEERING,2107,282415.700,02000000,471d,15824;INS_ALIGNMENT_COMPLETE,INS_RTKFIXED,37.37048807554,126.72451000285,11.3689,22.3000,-0.1889,0.2508,0.0038,-0.308402860,1.363313459,120.035668332,0.4468,0.2975,0.5625,0.1152,0.0938,0.0768,0.1401,0.1449,5.0346,0f000001,0*269cbb1b\n\t", "INSPVAXA,USB3,0,49.5,FINESTEERING,2107,282416.200,02000000,471d,15824;INS_ALIGNMENT_COMPLETE,INS_RTKFIXED,37.37048732666,126.72451132645,11.3727,22.3000,-0.2024,0.2646,0.0068,-0.344354829,1.559210135,120.006452776,0.4418,0.2949,0.5567,0.1151,0.0940,0.0765,0.1400,0.1448,5.0344,0f000001,0*5f55c88e\n\t", "INSPVAXA,USB3,0,49.5,FINESTEERING,2107,282416.700,02000000,471d,15824;INS_ALIGNMENT_COMPLETE,INS_RTKFIXED,37.37048655948,126.72451266499,11.3766,22.3000,-0.1941,0.2563,0.0061,-0.377791585,1.578777969,120.002147142,0.4418,0.2949,0.5567,0.1151,0.0940,0.0765,0.1400,0.1448,5.0344,0f000001,0*34897afe\n\t", "INSPVAXA,USB3,0,52.5,FINESTEERING,2107,282417.700,02000000,471d,15824;INS_ALIGNMENT_COMPLETE,INS_RTKFIXED,37.37048504382,126.72451529790,11.3842,22.3000,-0.1953,0.2454,0.0181,-0.246271614,1.533033405,119.744385532,0.4392,0.2938,0.5521,0.1151,0.0941,0.0764,0.1399,0.1448,5.0342,0f000001,0*775a7cde\n\t", "INSPVAXA,USB3,0,49.5,FINESTEERING,2107,282418.200,02000000,471d,15824;INS_ALIGNMENT_COMPLETE,INS_RTKFIXED,37.37048430161,126.72451659682,11.3895,22.3000,-0.1860,0.2574,0.0118,-0.194523398,1.357517182,119.541638486,0.4391,0.2937,0.5490,0.1153,0.0938,0.0764,0.1398,0.1447,5.0342,0f000001,0*fd6a5a6b\n\t", "INSPVAXA,USB3,0,49.5,FINESTEERING,2107,282418.700,02000000,471d,15824;INS_ALIGNMENT_COMPLETE,INS_RTKFIXED,37.37048357095,126.72451792235,11.3949,22.3000,-0.1880,0.2631,0.0129,-0.293493198,1.431848983,119.317686848,0.4391,0.2937,0.5490,0.1153,0.0938,0.0764,0.1398,0.1447,5.0342,0f000001,0*f85c4eed\n\t", "INSPVAXA,USB3,0,51.5,FINESTEERING,2107,282419.200,02000000,471d,15824;INS_ALIGNMENT_COMPLETE,INS_RTKFIXED,37.37048282849,126.72451926994,11.3994,22.3000,-0.1790,0.2403,0.0146,-0.323412826,1.420573693,119.067840661,0.4387,0.2935,0.5464,0.1153,0.0936,0.0764,0.1397,0.1447,5.0349,0f000001,0*dfe7d2ed\n\t", "INSPVAXA,USB3,0,51.5,FINESTEERING,2107,282419.700,02000000,471d,15824;INS_ALIGNMENT_COMPLETE,INS_RTKFIXED,37.37048208962,126.72452059781,11.4036,22.3000,-0.1738,0.2412,0.0141,-0.294957453,1.425673265,118.815782482,0.4387,0.2935,0.5464,0.1153,0.0936,0.0764,0.1397,0.1447,5.0349,0f000001,0*b9942f72\n\t", "INSPVAXA,USB3,0,50.5,FINESTEERING,2107,282420.200,02000000,471d,15824;INS_ALIGNMENT_COMPLETE,INS_RTKFIXED,37.37048136193,126.72452192165,11.4068,22.3000,-0.1787,0.2514,0.0118,-0.301136981,1.598998965,118.572497576,0.4423,0.2941,0.5460,0.1156,0.0933,0.0766,0.1396,0.1447,5.0359,0f000001,0*0dbcadaf\n\t", "INSPVAXA,USB3,0,50.5,FINESTEERING,2107,282420.700,02000000,471d,15824;INS_ALIGNMENT_COMPLETE,INS_RTKFIXED,37.37048063557,126.72452326406,11.4104,22.3000,-0.1682,0.2469,0.0144,-0.349485700,1.489707131,118.312804770,0.4423,0.2941,0.5460,0.1156,0.0933,0.0766,0.1396,0.1447,5.0359,0f000001,0*9bf849d5\n\t", "INSPVAXA,USB3,0,48.0,FINESTEERING,2107,282421.200,02000000,471d,15824;INS_ALIGNMENT_COMPLETE,INS_RTKFIXED,37.37047991282,126.72452459987,11.4134,22.3000,-0.1640,0.2507,0.0070,-0.436089069,1.502424265,118.039794860,0.4455,0.2944,0.5457,0.1157,0.0930,0.0767,0.1395,0.1446,5.0372,0f000001,0*71ca6260\n\t", "INSPVAXA,USB3,0,48.0,FINESTEERING,2107,282421.700,02000000,471d,15824;INS_ALIGNMENT_COMPLETE,INS_RTKFIXED,37.37047920210,126.72452588480,11.4143,22.3000,-0.1661,0.2579,0.0075,-0.445939557,1.526205768,117.767448761,0.4455,0.2944,0.5457,0.1157,0.0930,0.0767,0.1395,0.1446,5.0372,0f000001,0*bff7dfe5\n\t", "INSPVAXA,USB3,0,52.0,FINESTEERING,2107,282422.200,02000000,471d,15824;INS_ALIGNMENT_COMPLETE,INS_RTKFIXED,37.37047849051,126.72452721632,11.4160,22.3000,-0.1641,0.2604,0.0088,-0.542046801,1.417066343,117.580039835,0.4474,0.2945,0.5457,0.1156,0.0927,0.0768,0.1395,0.1446,5.0385,0f000001,0*5a4f325f\n\t", "INSPVAXA,USB3,0,52.0,FINESTEERING,2107,282422.700,02000000,471d,15824;INS_ALIGNMENT_COMPLETE,INS_RTKFIXED,37.37047779147,126.72452855561,11.4180,22.3000,-0.1674,0.2510,0.0061,-0.538633427,1.577251598,117.409835923,0.4474,0.2945,0.5457,0.1156,0.0927,0.0768,0.1395,0.1446,5.0385,0f000001,0*702f4b29\n\t", "INSPVAXA,USB3,0,53.0,FINESTEERING,2107,282423.200,02000000,471d,15824;INS_ALIGNMENT_COMPLETE,INS_RTKFIXED,37.37047709132,126.72452988330,11.4199,22.3000,-0.1693,0.2361,0.0114,-0.484097590,1.645236384,117.249213535,0.4481,0.2944,0.5459,0.1153,0.0924,0.0769,0.1394,0.1445,5.0397,0f000001,0*1f110da8\n\t", "INSPVAXA,USB3,0,53.0,FINESTEERING,2107,282423.700,02000000,471d,15824;INS_ALIGNMENT_COMPLETE,INS_RTKFIXED,37.37047638174,126.72453122858,11.4229,22.3000,-0.1794,0.2589,0.0063,-0.583943678,1.497224393,117.186202901,0.4481,0.2944,0.5459,0.1153,0.0924,0.0769,0.1394,0.1445,5.0397,0f000001,0*d1d8ac53\n\t", "INSPVAXA,USB3,0,47.5,FINESTEERING,2107,282424.200,02000000,471d,15824;INS_ALIGNMENT_COMPLETE,INS_RTKFIXED,37.37047566683,126.72453256018,11.4256,22.3000,-0.1669,0.2594,-0.0024,-0.470106549,1.538680379,117.122704089,0.4483,0.2943,0.5461,0.1150,0.0923,0.0770,0.1394,0.1445,5.0409,0f000001,0*dc6910b4\n\t", "INSPVAXA,USB3,0,47.5,FINESTEERING,2107,282424.700,02000000,471d,15824;INS_ALIGNMENT_COMPLETE,INS_RTKFIXED,37.37047494841,126.72453391705,11.4289,22.3000,-0.1673,0.2511,-0.0021,-0.336586213,1.463245271,117.104928251,0.4483,0.2943,0.5461,0.1150,0.0923,0.0770,0.1394,0.1445,5.0409,0f000001,0*1c6dfd0e\n\t", "INSPVAXA,USB3,0,52.5,FINESTEERING,2107,282425.200,02000000,471d,15824;INS_ALIGNMENT_COMPLETE,INS_RTKFIXED,37.37047424170,126.72453526540,11.4324,22.3000,-0.1767,0.2603,-0.0045,-0.387302146,1.336492111,117.087271319,0.4481,0.2942,0.5464,0.1148,0.0922,0.0770,0.1394,0.1445,5.0421,0f000001,0*5b1ecf9b\n\t", "INSPVAXA,USB3,0,52.5,FINESTEERING,2107,282425.700,02000000,471d,15824;INS_ALIGNMENT_COMPLETE,INS_RTKFIXED,37.37047353381,126.72453661330,11.4355,22.3000,-0.1756,0.2651,-0.0041,-0.429146495,1.196465105,117.112616572,0.4481,0.2942,0.5464,0.1148,0.0922,0.0770,0.1394,0.1445,5.0421,0f000001,0*c119c68d\n\t", "INSPVAXA,USB3,0,49.0,FINESTEERING,2107,282426.200,02000000,471d,15824;INS_ALIGNMENT_COMPLETE,INS_RTKFIXED,37.37047281927,126.72453797131,11.4379,22.3000,-0.1734,0.2394,0.0077,-0.416203988,1.155690665,117.100710288,0.4473,0.2939,0.5465,0.1146,0.0922,0.0771,0.1395,0.1444,5.0432,0f000001,0*775443d5\n\t", "INSPVAXA,USB3,0,49.0,FINESTEERING,2107,282426.700,02000000,471d,15824;INS_ALIGNMENT_COMPLETE,INS_RTKFIXED,37.37047210734,126.72453930572,11.4405,22.3000,-0.1867,0.2504,0.0028,-0.209968626,1.098729863,117.099023809,0.4473,0.2939,0.5465,0.1146,0.0922,0.0771,0.1395,0.1444,5.0432,0f000001,0*f26e42b0\n\t", "INSPVAXA,USB3,0,49.0,FINESTEERING,2107,282427.200,02000000,471d,15824;INS_ALIGNMENT_COMPLETE,INS_RTKFIXED,37.37047139601,126.72454064039,11.4416,22.3000,-0.1731,0.2492,-0.0012,-0.127511151,0.940148188,117.168833754,0.4465,0.2938,0.5466,0.1144,0.0924,0.0771,0.1395,0.1444,5.0441,0f000001,0*6d877c07\n\t", "INSPVAXA,USB3,0,49.0,FINESTEERING,2107,282427.700,02000000,471d,15824;INS_ALIGNMENT_COMPLETE,INS_RTKFIXED,37.37047069525,126.72454194730,11.4442,22.3000,-0.1701,0.2495,0.0012,-0.095196200,0.956873575,117.185221868,0.4465,0.2938,0.5466,0.1144,0.0924,0.0771,0.1395,0.1444,5.0441,0f000001,0*84a20544\n\t", "INSPVAXA,USB3,0,48.5,FINESTEERING,2107,282428.200,02000000,471d,15824;INS_ALIGNMENT_COMPLETE,INS_RTKFIXED,37.37046998613,126.72454328070,11.4463,22.3000,-0.1686,0.2345,-0.0007,-0.178803832,1.054572060,117.268598245,0.4452,0.2937,0.5465,0.1143,0.0923,0.0771,0.1395,0.1444,5.0443,0f000001,0*71fff611\n\t", "INSPVAXA,USB3,0,48.5,FINESTEERING,2107,282428.700,02000000,471d,15824;INS_ALIGNMENT_COMPLETE,INS_RTKFIXED,37.37046928771,126.72454456958,11.4489,22.3000,-0.1768,0.2502,0.0012,-0.177631825,1.040630154,117.335486579,0.4452,0.2937,0.5465,0.1143,0.0923,0.0771,0.1395,0.1444,5.0443,0f000001,0*5554e59a\n\t", "INSPVAXA,USB3,0,50.5,FINESTEERING,2107,282429.200,02000000,471d,15824;INS_ALIGNMENT_COMPLETE,INS_RTKFIXED,37.37046858218,126.72454587294,11.4510,22.3000,-0.1735,0.2382,-0.0057,-0.224101923,1.178682503,117.429703451,0.4445,0.2937,0.5467,0.1141,0.0923,0.0771,0.1395,0.1444,5.0440,0f000001,0*7240883e\n\t", "INSPVAXA,USB3,0,50.5,FINESTEERING,2107,282429.700,02000000,471d,15824;INS_ALIGNMENT_COMPLETE,INS_RTKFIXED,37.37046786468,126.72454718856,11.4534,22.3000,-0.1761,0.2406,-0.0007,-0.208083401,1.502280948,117.509973758,0.4445,0.2937,0.5467,0.1141,0.0923,0.0771,0.1395,0.1444,5.0440,0f000001,0*e6f82928\n\t", "INSPVAXA,USB3,0,50.5,FINESTEERING,2107,282430.200,02000000,471d,15824;INS_ALIGNMENT_COMPLETE,INS_RTKFIXED,37.37046713454,126.72454853223,11.4571,22.3000,-0.1871,0.2437,0.0106,-0.235134263,1.524805783,117.657150999,0.4436,0.2937,0.5464,0.1140,0.0923,0.0770,0.1395,0.1444,5.0440,0f000001,0*40fb5b15\n\t", "INSPVAXA,USB3,0,50.5,FINESTEERING,2107,282430.700,02000000,471d,15824;INS_ALIGNMENT_COMPLETE,INS_RTKFIXED,37.37046640925,126.72454987215,11.4613,22.3000,-0.1820,0.2459,0.0096,-0.221423575,1.571464765,117.878951435,0.4436,0.2937,0.5464,0.1140,0.0923,0.0770,0.1395,0.1444,5.0440,0f000001,0*a08ac800\n\t", "INSPVAXA,USB3,0,50.5,FINESTEERING,2107,282431.200,02000000,471d,15824;INS_ALIGNMENT_COMPLETE,INS_RTKFIXED,37.37046567554,126.72455119637,11.4651,22.3000,-0.1719,0.2427,0.0197,-0.166037834,1.730159075,118.106300451,0.4429,0.2934,0.5460,0.1140,0.0922,0.0770,0.1395,0.1444,5.0446,0f000001,0*c5fa0f53\n\t", "INSPVAXA,USB3,0,50.5,FINESTEERING,2107,282431.700,02000000,471d,15824;INS_ALIGNMENT_COMPLETE,INS_RTKFIXED,37.37046493957,126.72455254233,11.4688,22.3000,-0.1743,0.2458,0.0116,-0.329831590,1.590746400,118.317737739,0.4429,0.2934,0.5460,0.1140,0.0922,0.0770,0.1395,0.1444,5.0446,0f000001,0*f79436a0\n\t", "INSPVAXA,USB3,0,51.5,FINESTEERING,2107,282432.200,02000000,471d,15824;INS_ALIGNMENT_COMPLETE,INS_RTKFIXED,37.37046419639,126.72455389364,11.4732,22.3000,-0.1776,0.2446,0.0108,-0.495947229,1.503105474,118.571137499,0.4424,0.2936,0.5455,0.1139,0.0922,0.0769,0.1394,0.1444,5.0458,0f000001,0*be714efa\n\t", "INSPVAXA,USB3,0,51.5,FINESTEERING,2107,282432.700,02000000,471d,15824;INS_ALIGNMENT_COMPLETE,INS_RTKFIXED,37.37046345455,126.72455522466,11.4784,22.3000,-0.1781,0.2428,0.0084,-0.542024872,1.613123448,118.821399108,0.4424,0.2936,0.5455,0.1139,0.0922,0.0769,0.1394,0.1444,5.0458,0f000001,0*f6f3aed6\n\t", "INSPVAXA,USB3,0,50.0,FINESTEERING,2107,282433.200,02000000,471d,15824;INS_ALIGNMENT_COMPLETE,INS_RTKFIXED,37.37046270348,126.72455655878,11.4838,22.3000,-0.1795,0.2457,0.0085,-0.467602875,1.636327980,119.061626525,0.4415,0.2938,0.5451,0.1139,0.0923,0.0769,0.1394,0.1444,5.0472,0f000001,0*8d27345e\n\t", "DUALANTENNAHEADINGA,USB3,0,50.0,FINESTEERING,2107,282433.700,02000000,d426,15824;SOL_COMPUTED,NARROW_FLOAT,-1.000000000,131.824783325,-60.644287109,0.0,360.000000000,180.000000000,\"631T\",16,7,7,6,04,00,20,03*5e82c6fa\n\t", "INSPVAXA,USB3,0,51.0,FINESTEERING,2107,282434.200,02000000,471d,15824;INS_ALIGNMENT_COMPLETE,INS_RTKFIXED,37.37046121342,126.72455921489,11.4947,22.3000,-0.1798,0.2490,0.0001,-0.438174613,1.842528382,119.643730072,0.4410,0.2940,0.5447,0.1139,0.0923,0.0769,0.1394,0.1443,5.0488,0f000001,0*2736b416\n\t", "DUALANTENNAHEADINGA,USB3,0,51.0,FINESTEERING,2107,282434.700,02000000,d426,15824;SOL_COMPUTED,NARROW_FLOAT,-1.000000000,123.396003723,-59.946563721,0.0,360.000000000,180.000000000,\"631T\",18,7,7,6,04,00,20,03*e2309186\n\t", "INSPVAXA,USB3,0,52.0,FINESTEERING,2107,282435.200,02000000,471d,15824;INS_ALIGNMENT_COMPLETE,INS_RTKFIXED,37.37045967232,126.72456187341,11.5062,22.3000,-0.1775,0.2335,0.0126,-0.320080910,1.572819973,120.246717938,0.4403,0.2940,0.5441,0.1137,0.0923,0.0768,0.1394,0.1443,5.0504,0f000001,0*2715df5d\n\t", "INSPVAXA,USB3,0,52.0,FINESTEERING,2107,282435.700,02000000,471d,15824;INS_ALIGNMENT_COMPLETE,INS_RTKFIXED,37.37045891592,126.72456315232,11.5133,22.3000,-0.1801,0.2388,0.0143,-0.294831475,1.595184630,120.686846518,0.4403,0.2940,0.5441,0.1137,0.0923,0.0768,0.1394,0.1443,5.0504,0f000001,0*d40acedf\n\t", "DUALANTENNAHEADINGA,USB3,0,49.0,FINESTEERING,2107,282436.200,02000000,d426,15824;SOL_COMPUTED,L1_FLOAT,-1.000000000,106.640296936,-71.318817139,0.0,360.000000000,180.000000000,\"631T\",16,6,6,6,04,00,20,02*b4f0dd4d\n\t", "INSPVAXA,USB3,0,49.0,FINESTEERING,2107,282436.700,02000000,471d,15824;INS_ALIGNMENT_COMPLETE,INS_RTKFIXED,37.37045734595,126.72456573410,11.5280,22.3000,-0.1935,0.2298,0.0134,-0.155063449,1.404576364,121.642005651,0.4395,0.2941,0.5437,0.1137,0.0923,0.0768,0.1394,0.1443,5.0520,0f000001,0*bb2e31e4\n\t", "DUALANTENNAHEADINGA,USB3,0,50.0,FINESTEERING,2107,282437.200,02000000,d426,15824;SOL_COMPUTED,L1_FLOAT,-1.000000000,96.910743713,-72.679077148,0.0,360.000000000,180.000000000,\"631T\",19,6,6,6,04,00,20,02*8360ff91\n\t", "INSPVAXA,USB3,0,50.0,FINESTEERING,2107,282437.700,02000000,471d,15824;INS_ALIGNMENT_COMPLETE,INS_RTKFIXED,37.37045573344,126.72456827532,11.5401,22.3000,-0.1925,0.2230,0.0039,-0.101664053,1.395103847,122.819960781,0.4390,0.2940,0.5434,0.1136,0.0923,0.0768,0.1393,0.1443,5.0536,0f000001,0*7037bf1b\n\t", "INSPVAXA,USB3,0,50.0,FINESTEERING,2107,282438.200,02000000,471d,15824;INS_ALIGNMENT_COMPLETE,INS_RTKFIXED,37.37045491060,126.72456953243,11.5455,22.3000,-0.2008,0.2357,0.0053,0.014344275,1.355437453,123.346628191,0.4390,0.2941,0.5434,0.1137,0.0924,0.0768,0.1393,0.1442,5.0551,0f000001,0*dff132ba\n\t", "DUALANTENNAHEADINGA,USB3,0,50.0,FINESTEERING,2107,282438.700,02000000,d426,15824;SOL_COMPUTED,L1_FLOAT,-1.000000000,88.413047791,-71.788269043,0.0,360.000000000,180.000000000,\"631T\",18,6,6,6,04,00,20,02*2c629dff\n\t", "INSPVAXA,USB3,0,50.0,FINESTEERING,2107,282439.200,02000000,471d,15824;INS_ALIGNMENT_COMPLETE,INS_RTKFIXED,37.37045327515,126.72457200687,11.5547,22.3000,-0.1947,0.2312,0.0176,0.007839665,1.196473150,124.504878880,0.4394,0.2943,0.5435,0.1138,0.0925,0.0768,0.1393,0.1442,5.0565,0f000001,0*62131131\n\t", "INSPVAXA,USB3,0,50.0,FINESTEERING,2107,282439.700,02000000,471d,15824;INS_ALIGNMENT_COMPLETE,INS_RTKFIXED,37.37045245095,126.72457319458,11.5591,22.3000,-0.1909,0.2308,0.0250,0.014196005,1.345300679,124.975912941,0.4394,0.2943,0.5435,0.1138,0.0925,0.0768,0.1393,0.1442,5.0565,0f000001,0*c01a2c95\n\t", "DUALANTENNAHEADINGA,USB3,0,50.5,FINESTEERING,2107,282440.200,02000000,d426,15824;SOL_COMPUTED,L1_FLOAT,-1.000000000,104.733528137,-71.981353760,0.0,360.000000000,180.000000000,\"631T\",16,6,6,6,04,00,20,02*496cf2b0\n\t", "INSPVAXA,USB3,0,50.5,FINESTEERING,2107,282440.700,02000000,471d,15824;INS_ALIGNMENT_COMPLETE,INS_RTKFIXED,37.37045078135,126.72457562131,11.5665,22.3000,-0.1912,0.2138,0.0152,-0.119688285,1.522549253,125.693506579,0.4396,0.2937,0.5434,0.1139,0.0925,0.0768,0.1392,0.1442,5.0578,0f000001
